vi "VISA_session_open.vi"(8 "error in (no error)":errorcluster, 11 "VISA resource name":refnum<visa-resource-name>) -> (0 "error out":errorcluster, 3 "VISA resource name out":refnum<visa-resource-name>)   [LabVIEW 2015]
doc: "This VI opens VISA port"
panel:
  # "This is valid for both:\n19572 & 19052"
  # "Open port"
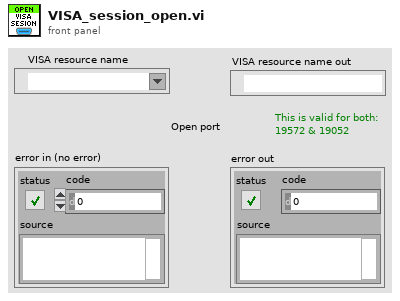
[diagram p1: front panel]
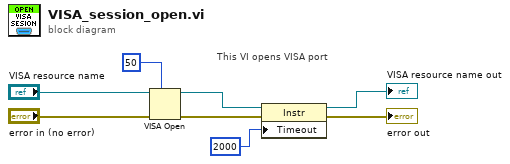
[diagram p0: block diagram]
diagram:
  # "This VI opens VISA port"
  n1 = VISA Open(timeout (0)=u32 50 ("VISA Open timeout (0)"), error in (no error)="error in (no error)", VISA resource name="VISA resource name") -> (VISA resource name=w4:refnum<visa-resource-name>, error out=w3:errorcluster)  [unwired: 2 in]
  n2 = property class="Instr"(reference=w4, error in=w3, "Timeout"=u32 2000) -> (reference out=→"VISA resource name out":refnum<visa-resource-name>, error out=→"error out":errorcluster)
